vi "Teleop.vi"(10 "Match Info":T5={"Autonomous Elapsed Seconds"=0.0, "TeleOp Elapsed Seconds"=0.0, "Disabled Elapsed Seconds"=0.0, "Visited Autonomous"=FALSE, "Visited TeleOp"=FALSE, "Visited Disabled"=FALSE, "Autonomous Settings"={"Autonomous Style"=enum."Independent", "VI Refnum"=refnum}}, 11 "Call Context":T6) -> ()   [LabVIEW 2016]
doc: "This VI is called for each TeleOp packet received from the DS where the robot is not disabled. It is often used to read from the joysticks and update I/O or to update setpoints for timed control loops. It should complete and return within 20 milliseconds or it may miss DS packets."
uses:
  <vilib>/Rock Robotics/WPI/DriverStation/WPI_DriverStationDerivedRobotMode.ctl
  <vilib>/Rock Robotics/WPI/DriverStation/WPI_DriverStationMatch Info.ctl
  <vilib>/Rock Robotics/WPI/Relay/WPI_RelayValue.ctl
  <vilib>/Rock Robotics/WPI/Solenoid/WPI_SolenoidValue.ctl
  <vilib>/Rock Robotics/WPI/Utilities/WPI_GetSetVariantRefNum.vi
  <vilib>/Rock Robotics/Network Tables/NT Write Boolean Array.vi
  <vilib>/Rock Robotics/Network Tables/NT Write Numeric Array.vi
  <vilib>/Rock Robotics/Network Tables/NT Read Boolean.vi
  <vilib>/Rock Robotics/Network Tables/NT Read Number.vi
  <vilib>/Rock Robotics/WPI/Solenoid/WPI_SolenoidSetEnum.vi
  <vilib>/Rock Robotics/Network Tables/NT Write Number.vi
  Robot Global Data - Test.vi
  <vilib>/addons/control/pid/pid.llb/PID (DBL).vi
  <vilib>/Rock Robotics/WPI/RobotDrive/WPI_RobotDriveMecanumDrive_Cartesian.vi
  <vilib>/addons/control/pid/NI_PID_pid.lvlib
  <vilib>/Rock Robotics/Network Tables/NT Write Boolean.vi
panel:
  out "Relay Toggle Output":bool
  out "RelayValue":T1
  out "Compressor Running":bool
  out "Enabled":bool
  out "Raw Out Left":cluster{dbl, dbl}(graph)={0.03662109, 0.056152338}
  out "Raw Out Right":cluster{dbl, dbl}(graph)={0.0288085908, 0.026855466}
  out "Average of Right Infrared":cluster{dbl, dbl}(graph)={2232.752755466602, 2291.2959364383637}
  out "Average of Left Infrared":cluster{dbl, dbl}(graph)={1983.0102786129094, 926.8937522387996}
  out "error out":errorcluster
  out "PSI":dbl(knob) scale=0.0..200.0
  out "Average of Right Ultrasonic":cluster{dbl, dbl}(graph)={2232.752755466602, 2291.2959364383637}
  out "Average of Left Ultrasonic":cluster{dbl, dbl}(graph)={1983.0102786129094, 926.8937522387996}
  in  "climberpower":dbl(slide)=0.3 scale=0.0..1.0
  in  "deadband thing":dbl=0.13
  in  "Strafe":dbl(slide)=1.0 caption="Strafe Scale" scale=0.0..1.0
  in  "Deadband":dbl(slide)=0.10404624277456642 scale=-1.0..1.0
  out "useless data point LOL":dbl=-2.99
  out "derivative time (Td, min)":dbl
  out "integral time (Ti, min)":dbl=0.01
  out "proportional gain (Kc)":dbl=1.0
  in  "PID gains":T2={"proportional gain (Kc)"=1.0, "integral time (Ti, min)"=0.01, "derivative time (Td, min)"=0.0} {"derivative time (Td, min)" scale=0.0..0.05; "integral time (Ti, min)" scale=0.0..0.00243; "proportional gain (Kc)" scale=0.0..0.284195}
  in  "setpoint":dbl(slide) scale=-50.0..50.0
  out "Data":T3(graph)={"setpoint"=0.0, "Yaw"=-2.99, "dt out (s)"=0.018000000854954123}
  out "Yaw":dbl=-2.99
  out "YRPHfH 2":T4={"Yaw"=-2.99, "Roll"=1.62, "Pitch"=0.41, "Heading"=0.0, "Fused Heading"=357.0}
  out "Sample Slider 1":dbl(slide) scale=0.0..5.0
  out "Sample Boolean 3":bool
  out "Sample Boolean 2":bool
  in  "Match Info 2":T5={"Autonomous Elapsed Seconds"=0.0, "TeleOp Elapsed Seconds"=24.241, "Disabled Elapsed Seconds"=0.519, "Visited Autonomous"=FALSE, "Visited TeleOp"=TRUE, "Visited Disabled"=TRUE, "Autonomous Settings"={"Autonomous Style"=enum."Independent", "VI Refnum"=refnum}}
  in  "Call Context 2":T6=enum."Stop"
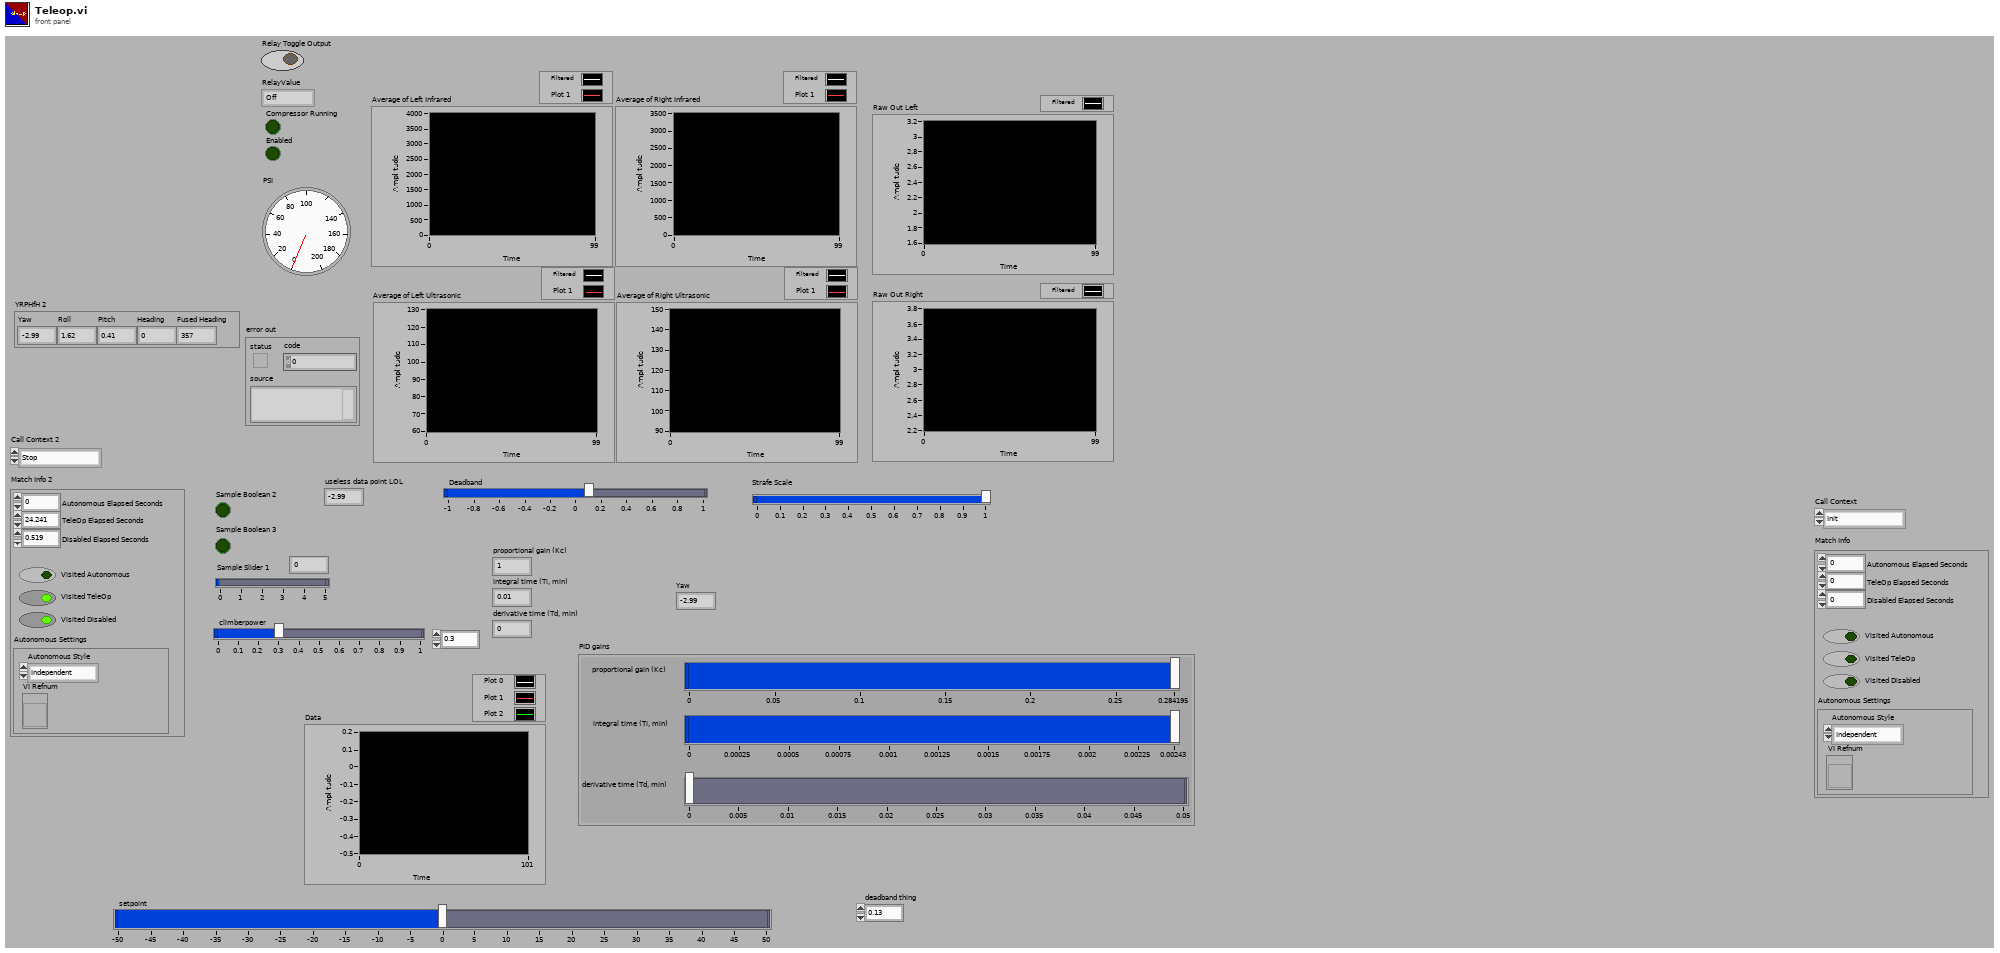
[diagram p1: front panel]
types:
  T1 = typedef "WPI_RelayValue.ctl" = enum16{"Off", "On", "Forward", "Reverse"}
  T2 = cluster{"proportional gain (Kc)":dbl, "integral time (Ti, min)":dbl, "derivative time (Td, min)":dbl}
  T3 = cluster{"setpoint":dbl, "Yaw":dbl, "dt out (s)":dbl}
  T4 = cluster{"Yaw":dbl, "Roll":dbl, "Pitch":dbl, "Heading":dbl, "Fused Heading":dbl}
  T5 = typedef "WPI_DriverStationMatch Info.ctl" = cluster{"Autonomous Elapsed Seconds":dbl, "TeleOp Elapsed Seconds":dbl, "Disabled Elapsed Seconds":dbl, "Visited Autonomous":bool, "Visited TeleOp":bool, "Visited Disabled":bool, "Autonomous Settings":cluster{"Autonomous Style":enum16{"Iterative", "Independent"}, "VI Refnum":refnum<vi>}}
  T6 = typedef "WPI_DriverStationDerivedRobotMode.ctl" = enum16{"Init", "Execute", "Stop"}
  T7 = typedef "WPI_SolenoidValue.ctl" = enum16{"Off", "On", "Forward", "Reverse"}
  T8 = typedef "WPI_AnalogChannelDevRef.ctl" = cluster{"DevStatus":errorcluster, "Analog Channel":T9}
  T9 = typedef "FPGA_AIChannel.ctl" = enum8{"AI 0", "AI 1", "AI 2", "AI 3", "AI MXP 0", "AI MXP 1", "AI MXP 2", "AI MXP 3", "Invalid"}
  T10 = typedef "WPI_CompressorDevRef.ctl" = cluster{"DevStatus":errorcluster, "Pneumatics Control Module":u8}
  T11 = typedef "WPI_RelayDevRef.ctl" = cluster{"DevStatus":errorcluster, "Relay Channel":T12, "Relay Direction":T13}
  T12 = typedef "FPGA_DIORelayChannel.ctl" = enum8{"Relay 0", "Relay 1", "Relay 2", "Relay 3", "Invalid"}
  T13 = typedef "WPI_RelayDirection.ctl" = enum16{"Both directions", "Forward only", "Reverse only"}
  T14 = typedef "WPI_JoystickDevRef.ctl" = cluster{"Device":T15}
  T15 = typedef "WPI_JoystickDeviceEnum.ctl" = enum16{"USB 0", "USB 1", "USB 2", "USB 3", "USB 4", "USB 5"}
  T16 = typedef "WPI_MotorControlDeviceRef.ctl" = cluster{"DeviceStatus":errorcluster, "Type":T17, "PWM":cluster{"PWM Channel":T18, "DeadBand":T19}, "CAN":cluster{"Device Number":u8, "SetOutput VI Ref":variant, "GetOutput VI Ref":variant, "Enable VI Ref":variant, "Disable VI Ref":variant, "Data":variant}, "Invert":bool}
  T17 = typedef "WPI_MotorControlType.ctl" = enum16{"PWM", "CAN"}
  T18 = typedef "FPGA_DIOPWMChannel.ctl" = enum8{"PWM 0", "PWM 1", "PWM 2", "PWM 3", "PWM 4", "PWM 5", "PWM 6", "PWM 7", "PWM 8", "PWM 9", "PWM MXP 0", "PWM MXP 1", "PWM MXP 2", "PWM MXP 3", "PWM MXP 4", "PWM MXP 5", "PWM MXP 6", "PWM MXP 7", "PWM MXP 8", "PWM MXP 9", "Invalid"}
  T19 = typedef "WPI_PWMDeadband.ctl" = cluster{"Name":string, "maxPositivePwm":i32, "minPositivePwm":i32, "centerPwm":i32, "maxNegativePwm":i32, "minNegativePwm":i32, "angularRange":u16}
  T20 = typedef "WPI_SolenoidDevRef.ctl" = cluster{"DevStatus":errorcluster, "Pneumatics Control Module":u8, "Forward Solenoid Channel":T21, "Reverse Solenoid Channel":T21}
  T21 = typedef "WPI_SolenoidChannel.ctl" = enum8{"Solenoid 0", "Solenoid 1", "Solenoid 2", "Solenoid 3", "Solenoid 4", "Solenoid 5", "Solenoid 6", "Solenoid 7", "Invalid"}
  T22 = typedef "WPI_RobotDriveDevRef.ctl" = cluster{"DevStatus":errorcluster, "Motors[]":T16[], "Square Inputs":bool, "Max Output":dbl}
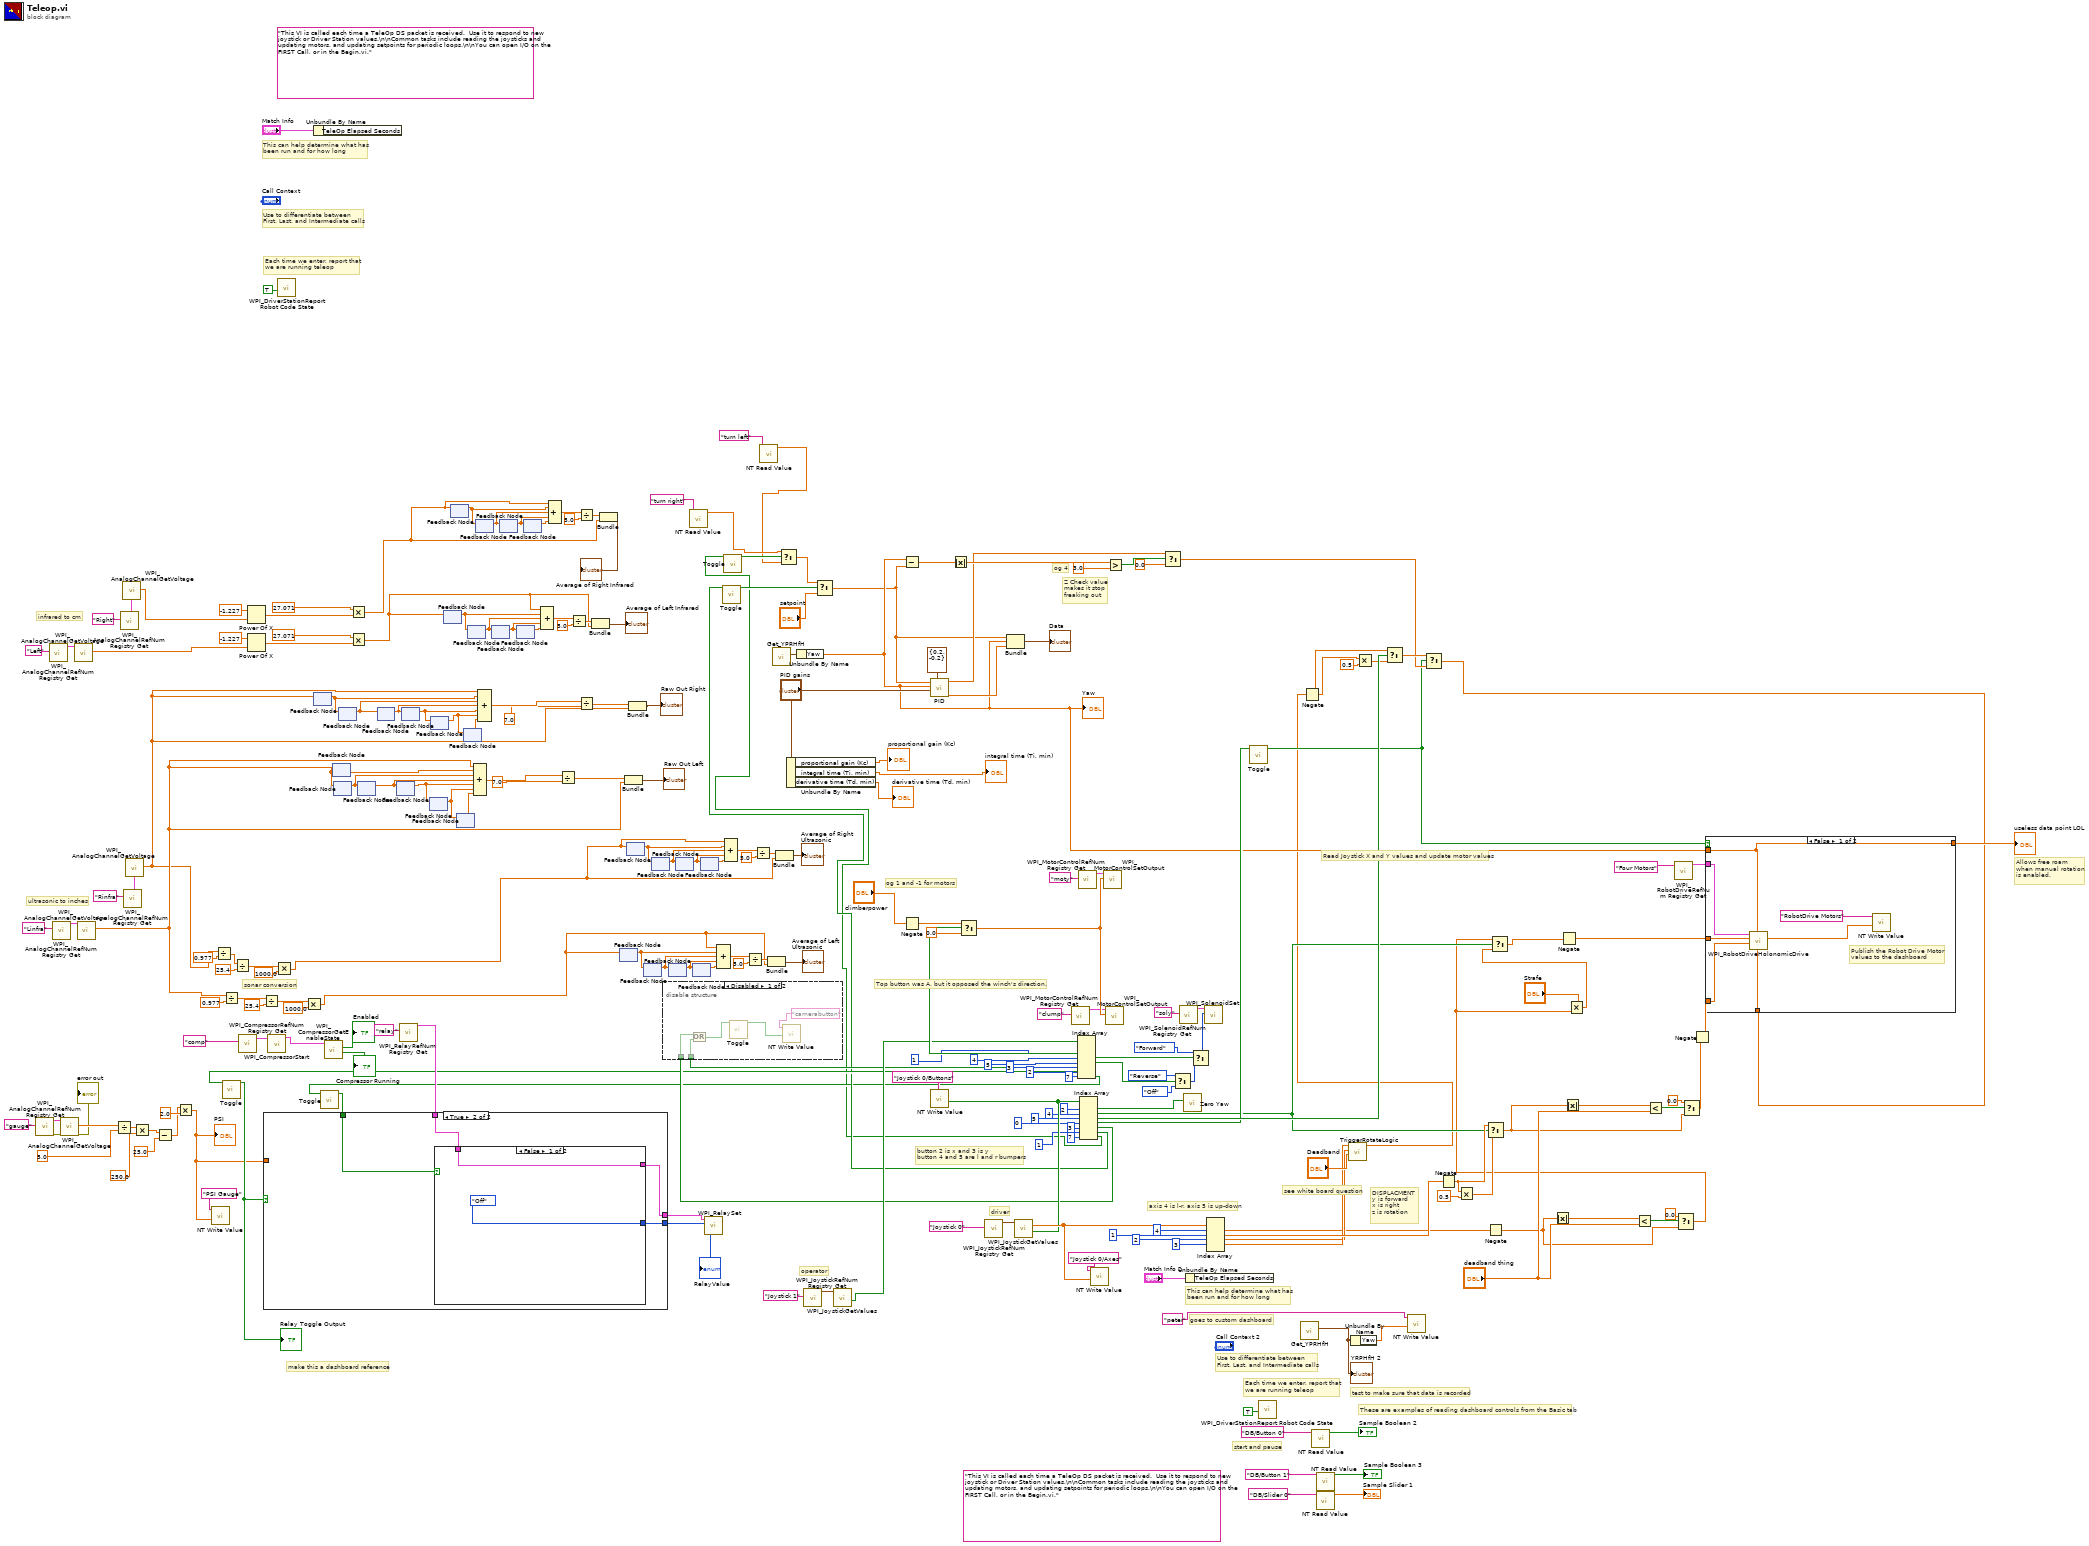
[diagram p0: block diagram]
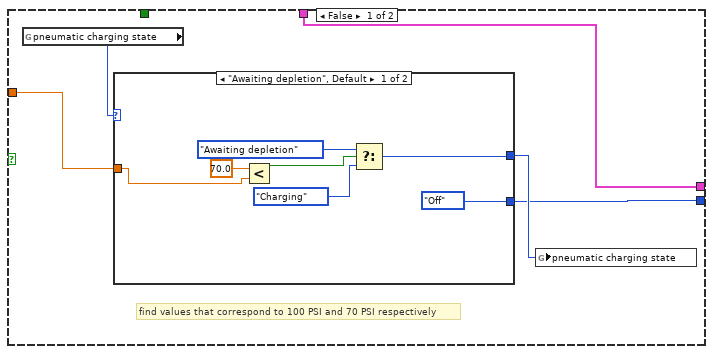
[diagram p2: hidden frame]
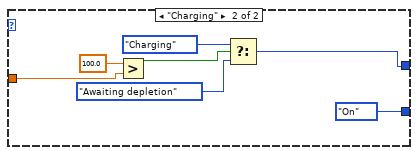
[diagram p3: hidden frame]
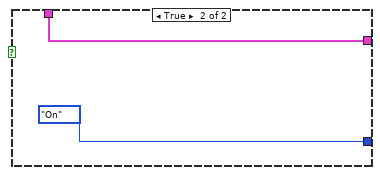
[diagram p4: hidden frame]
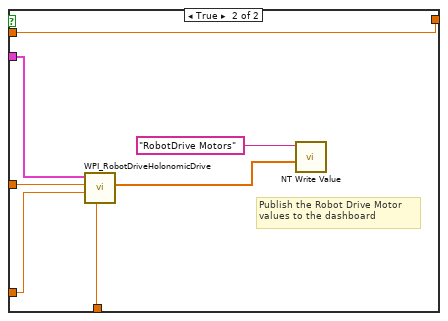
[diagram p6: hidden frame]
diagram:
  (unwired) "This VI is called each time a TeleOp DS packet is received.  Use it to respond to new joystick or Driver Station values.\n\nCommon tasks include reading the joysticks and updating motors, and updating setpoints for periodic loops.\n\nYou can open I/O on the FIRST Call, or in the Begin.vi."
  (unwired) "This VI is called each time a TeleOp DS packet is received.  Use it to respond to new joystick or Driver Station values.\n\nCommon tasks include reading the joysticks and updating motors, and updating setpoints for periodic loops.\n\nYou can open I/O on the FIRST Call, or in the Begin.vi."
  # "make this a dashboard reference"
  # "Top button was A, but it opposed the winch's direction."
  # "ultrasonic to inches"
  # "sonar conversion"
  # "infrared to cm"
  # "driver"
  # "operator"
  # "see white board question"
  # "axis 4 is l-r, axis 5 is up-down"
  # "og 1 and -1 for motors"
  # "og 4"
  # "Allows free roam\nwhen manual rotation\nis enabled."
  # "Z Check value\nmakes it stop\nfreaking out"
  # "start and pause"
  # "goes to custom dashboard"
  # "button 2 is x and 3 is y\nbutton 4 and 5 are l and r bumpers"
  # "DISPLACMENT\ny is forward\nx is right\nz is rotation"
  # "test to make sure that data is recorded"
  # "These are examples of reading dashboard controls from the Basic tab"
  # "Each time we enter, report that\nwe are running teleop"
  # "Use to differentiate between\nFirst, Last, and Intermediate calls"
  # "This can help determine what has\nbeen run and for how long"
  # "Read Joystick X and Y values and update motor values"
  # "Each time we enter, report that\nwe are running teleop"
  # "Use to differentiate between\nFirst, Last, and Intermediate calls"
  # "This can help determine what has\nbeen run and for how long"
  n1 = call <vilib>:"WPI_AnalogChannelRefNum Registry Get.vi"("refnum name"="gauge") -> ("error out"=w63:errorcluster, "AIDeviceRef"=w71:T8)  [unwired: 9 in]
  n2 = call <vilib>:"WPI_AnalogChannelRefNum Registry Get.vi"("refnum name"="Left") -> ("AIDeviceRef"=w46:T8)  [unwired: 9 in, 1 out]
  n3 = call <vilib>:"WPI_AnalogChannelRefNum Registry Get.vi"("refnum name"="Linfra") -> ("AIDeviceRef"=w128:T8)  [unwired: 9 in, 1 out]
  n4 = call <vilib>:"WPI_AnalogChannelGetVoltage.vi"("error in (no error)"=w63, "AIDeviceRef"=w71) -> ("error out"=→"error out":errorcluster, "Voltage"=w69:dbl)  [unwired: 7 in, 1 out]
  n5 = call <vilib>:"WPI_AnalogChannelGetVoltage.vi"("AIDeviceRef"=w46) -> ("Voltage"=w44:dbl)  [unwired: 8 in, 2 out]
  n6 = call <vilib>:"WPI_AnalogChannelGetVoltage.vi"("AIDeviceRef"=w128) -> ("Voltage"=w80:dbl)  [unwired: 8 in, 2 out]
  n7 = Divide(x=w69, y=5.0) -> (x/y=w68:dbl)
  n8 = call <vilib>:"WPI_AnalogChannelRefNum Registry Get.vi"("refnum name"="Right") -> ("AIDeviceRef"=w47:T8)  [unwired: 9 in, 1 out]
  n9 = call <vilib>:"WPI_AnalogChannelGetVoltage.vi"("AIDeviceRef"=w47) -> ("Voltage"=w45:dbl)  [unwired: 8 in, 2 out]
  n10 = call <vilib>:"WPI_AnalogChannelRefNum Registry Get.vi"("refnum name"="Rinfra") -> ("AIDeviceRef"=w129:T8)  [unwired: 9 in, 1 out]
  n11 = call <vilib>:"WPI_AnalogChannelGetVoltage.vi"("AIDeviceRef"=w129) -> ("Voltage"=w77:dbl)  [unwired: 8 in, 2 out]
  n12 = Multiply(x=w68, y=250.0) -> (x*y=w66:dbl)
  n13 = Subtract(x=w66, y=25.0) -> (x-y=w2:dbl)
  n14 = Multiply(x=w2, y=2.0) -> (x*y=w1:dbl)
  "PSI" <- w1
  n15 = call-poly <vilib>:"NT Write Value.vi"("Numeric"=w1, "Name"="PSI Gauge") -> ()  [unwired: 9 in, 1 out]
  n16 = Divide(x=w77, y=0.977) -> (x/y=w89:dbl)
  n17 = Divide(x=w80, y=0.977) -> (x/y=w83:dbl)
  n18 = Divide(x=w89, y=25.4) -> (x/y=w87:dbl)
  n19 = call <vilib>:"WPI_CompressorRefNum Registry Get.vi"("refnum name"="comp") -> ("CompressorDevRef"=w74:T10)  [unwired: 9 in, 1 out]
  n20 = Power Of X(1:w45, 2:-1.227 ("y")) -> (0:w41:dbl)
  n21 = Power Of X(1:w44, 2:-1.227 ("y")) -> (0:w40:dbl)
  n22 = Divide(x=w83, y=25.4) -> (x/y=w85:dbl)
  n23 = call <vilib>:"WPI_CompressorStart.vi"("CompressorDevRef"=w74) -> ("CompressorDevRef"=w6:T10)  [unwired: 9 in, 1 out]
  n24 = Multiply(x=w87, y=1000.0) -> (x*y=w81:dbl)
  n25 = call <vilib>:"WPI_DriverStationReport Robot Code State.vi"("TeleOp"=TRUE ("Autonomous")) -> ()  [unwired: 10 in, 1 out]
  n26 = Multiply(x=w85, y=1000.0) -> (x*y=w79:dbl)
  n27 = Unbundle By Name("Match Info") -> ()  [unwired: 1 out]
  n28 = feedback #1() -> (w103:dbl)  [unwired: 1 in]
  n29 = feedback-in #1(w77) -> ()
  n30 = call <vilib>:"WPI_CompressorGetEnableState.vi"("CompressorDevRef"=w6) -> ("Compressor Running"=→"Compressor Running":bool, "Enabled"=→"Enabled":bool)  [unwired: 7 in, 2 out]
  n31 = feedback #2() -> (w102:dbl)  [unwired: 1 in]
  n32 = feedback-in #2(w80) -> ()
  n33 = feedback #3() -> (w97:dbl)  [unwired: 1 in]
  n34 = feedback-in #3(w102) -> ()
  n35 = feedback #4() -> (w108:dbl)  [unwired: 1 in]
  n36 = feedback-in #4(w103) -> ()
  n37 = Multiply(x=27.071, y=w41) -> (x*y=w22:dbl)
  n38 = Multiply(x=27.071, y=w40) -> (x*y=w23:dbl)
  n39 = feedback #5() -> (w101:dbl)  [unwired: 1 in]
  n40 = feedback-in #5(w97) -> ()
  n41 = feedback #6() -> (w104:dbl)  [unwired: 1 in]
  n42 = feedback-in #6(w108) -> ()
  n43 = feedback #7() -> (w96:dbl)  [unwired: 1 in]
  n44 = feedback-in #7(w101) -> ()
  n45 = call <vilib>:"WPI_RelayRefNum Registry Get.vi"("refnum name"="relay") -> ("RelayDevRef"=w73:T11)  [unwired: 9 in, 1 out]
  n46 = feedback #8() -> (w93:dbl)  [unwired: 1 in]
  n47 = feedback-in #8(w104) -> ()
  n48 = feedback #9() -> (w95:dbl)  [unwired: 1 in]
  n49 = feedback-in #9(w96) -> ()
  n50 = feedback #10() -> (w92:dbl)  [unwired: 1 in]
  n51 = feedback-in #10(w93) -> ()
  n52 = feedback #11() -> (w37:dbl)  [unwired: 1 in]
  n53 = feedback-in #11(w23) -> ()
  n54 = feedback #12() -> (w24:dbl)  [unwired: 1 in]
  n55 = feedback-in #12(w22) -> ()
  n56 = feedback #13() -> (w94:dbl)  [unwired: 1 in]
  n57 = feedback-in #13(w95) -> ()
  n58 = feedback #14() -> (w91:dbl)  [unwired: 1 in]
  n59 = feedback-in #14(w92) -> ()
  n60 = feedback #15() -> (w36:dbl)  [unwired: 1 in]
  n61 = feedback-in #15(w37) -> ()
  n62 = Compound Arithmetic op=ADD(w80, w102, w97, w101, w96, w95, w94) -> (w98:dbl)
  n63 = feedback #16() -> (w30:dbl)  [unwired: 1 in]
  n64 = feedback-in #16(w24) -> ()
  n65 = Compound Arithmetic op=ADD(w77, w103, w108, w104, w93, w92, w91) -> (w107:dbl)
  n66 = feedback #17() -> (w31:dbl)  [unwired: 1 in]
  n67 = feedback-in #17(w36) -> ()
  n68 = feedback #18() -> (w25:dbl)  [unwired: 1 in]
  n69 = feedback-in #18(w30) -> ()
  n70 = feedback #19() -> (w32:dbl)  [unwired: 1 in]
  n71 = feedback-in #19(w31) -> ()
  n72 = feedback #20() -> (w26:dbl)  [unwired: 1 in]
  n73 = feedback-in #20(w25) -> ()
  n74 = Compound Arithmetic op=ADD(w23, w37, w36, w31, w32) -> (w35:dbl)
  n75 = Compound Arithmetic op=ADD(w22, w24, w30, w25, w26) -> (w29:dbl)
  n76 = Divide(x=w98, y=7.0) -> (x/y=w100:dbl)
  n77 = Divide(x=w35, y=5.0) -> (x/y=w33:dbl)
  n78 = Divide(x=w29, y=5.0) -> (x/y=w27:dbl)
  n79 = Divide(x=w107, y=7.0) -> (x/y=w105:dbl)
  n80 = Bundle(w33, w23) -> (→"Average of Left Infrared":cluster{dbl, dbl})  [unwired: 1 in]
  n81 = Bundle(w27, w22) -> (→"Average of Right Infrared":cluster{dbl, dbl})  [unwired: 1 in]
  n82 = feedback #21() -> (w124:dbl)  [unwired: 1 in]
  n83 = feedback-in #21(w79) -> ()
  n84 = Bundle(w100, "Voltage"=w80) -> (→"Raw Out Left":cluster{dbl, "Voltage":dbl})  [unwired: 1 in]
  n85 = feedback #22() -> (w110:dbl)  [unwired: 1 in]
  n86 = feedback-in #22(w81) -> ()
  n87 = Bundle(w105, "Voltage"=w77) -> (→"Raw Out Right":cluster{dbl, "Voltage":dbl})  [unwired: 1 in]
  n88 = feedback #23() -> (w123:dbl)  [unwired: 1 in]
  n89 = feedback-in #23(w124) -> ()
  n90 = feedback #24() -> (w116:dbl)  [unwired: 1 in]
  n91 = feedback-in #24(w110) -> ()
  n92 = feedback #25() -> (w117:dbl)  [unwired: 1 in]
  n93 = feedback-in #25(w123) -> ()
  n94 = feedback #26() -> (w111:dbl)  [unwired: 1 in]
  n95 = feedback-in #26(w116) -> ()
  n96 = call-poly <vilib>:"NT Read Value.vi"("Name"="turn right") -> ("Numeric"=w10:dbl)  [unwired: 9 in, 1 out]
  n97 = feedback #27() -> (w118:dbl)  [unwired: 1 in]
  n98 = feedback-in #27(w117) -> ()
  n99 = feedback #28() -> (w112:dbl)  [unwired: 1 in]
  n100 = feedback-in #28(w111) -> ()
  n101 = Compound Arithmetic op=ADD(w79, w124, w123, w117, w118) -> (w122:dbl)
  n102 = Compound Arithmetic op=ADD(w81, w110, w116, w111, w112) -> (w115:dbl)
  n103 = Divide(x=w122, y=5.0) -> (x/y=w120:dbl)
  n104 = Divide(x=w115, y=5.0) -> (x/y=w113:dbl)
  n105 = call-poly <vilib>:"NT Read Value.vi"("Name"="turn left") -> ("Numeric"=w9:dbl)  [unwired: 9 in, 1 out]
  n106 = Bundle(w120, w79) -> (→"Average of Left Ultrasonic":cluster{dbl, dbl})  [unwired: 1 in]
  n107 = call <vilib>:"Get_YPRHfH.vi"() -> ("YRPHfH"=w183:T4)  [unwired: 11 in]
  n108 = Bundle(w113, w81) -> (→"Average of Right Ultrasonic":cluster{dbl, dbl})  [unwired: 1 in]
  n109 = Unbundle By Name("PID gains") -> ("proportional gain (Kc)"=→"proportional gain (Kc)":dbl, "integral time (Ti, min)"=→"integral time (Ti, min)":dbl, "derivative time (Td, min)"=→"derivative time (Td, min)":dbl)
  n110 = Unbundle By Name(w183) -> ("Yaw"=w150:dbl)
  "Yaw" <- w150
  n111 = call <vilib>:"WPI_JoystickRefNum Registry Get.vi"("refnum name"="Joystick 1") -> ("JoystickDevRef"=w135:T14)  [unwired: 1 in, 9 out]
  n112 = call <vilib>:"WPI_JoystickGetValues.vi"("JoystickDevRef"=w135) -> ("Buttons"=w134:bool[])  [unwired: 6 in, 4 out]
  n113 = Negate(x="climberpower") -> (-x=w137:dbl)
  n114 = call <vilib>:"WPI_JoystickRefNum Registry Get.vi"("refnum name"="Joystick 0") -> ("JoystickDevRef"=w229:T14)  [unwired: 1 in, 9 out]
  n115 = call <vilib>:"WPI_JoystickGetValues.vi"("JoystickDevRef"=w229) -> ("Buttons"=w202:bool[], "Axes"=w226:dbl[])  [unwired: 6 in, 3 out]
  n116 = call-poly <vilib>:"NT Write Value.vi"("Boolean Array"=w202, "Name"="Joystick 0/Buttons") -> ()  [unwired: 9 in, 1 out]
  n117 = call <vilib>:"WPI_MotorControlRefNum Registry Get.vi"("refnum name"="clump") -> ("MotorControlDevRef"=w194:T16)  [unwired: 9 in, 1 out]
  n118 = Index Array(array=w134, index #2=1 ("index"), index #3=4 ("index"), index #4=5 ("index"), index #5=3 ("index"), index #6=2 ("index"), index #7=7 ("index")) -> (element #2=w215:bool, element #3=w157:bool, element #4=w155:bool, element #5=w127:bool, element #6=w56:bool, element #7=w14:bool)  [unwired: 1 in, 1 out]
  n119 = call "Toggle.vi"("Button Input"=w56) -> ("Toggle Output"=w16:bool)  [unwired: 9 in, 1 out]
  "Relay Toggle Output" <- w16
  n120 = call "Toggle.vi"("Button Input"=w14) -> ("Toggle Output"=w13:bool)  [unwired: 9 in, 1 out]
  n121 = case shown="True" w16 {
    tunnel: w73 -> [w237 w258]
    tunnel: w1 -> [w239 _]
    tunnel: w13 -> [_ w257]
    tunnel: [w237 w256] -> w8
    tunnel: [w236 w255] -> w7
    frame False {
      # "find values that correspond to 100 PSI and 70 PSI respectively"
      n122 = global read "Robot Global Data - Test.vi" "pneumatic charging state"() -> (w240:enum16{"Awaiting depletion", "Charging"})
      n123 = case shown="\"Awaiting depletion\", Default" w240 {
        tunnel: [WPI_RelayValue."Off" ("RelayValue") WPI_RelayValue."On" ("RelayValue")] -> w236
        tunnel: w239 -> [w242 w252]
        tunnel: [w241 w248] -> w238
        frame "Awaiting depletion", Default {
          n124 = Less?(x=70.0, y=w242) -> (x < y?=w245:bool)
          n125 = Select(t=enum16{"Awaiting depletion", "Charging"}."Awaiting depletion" ("pneumatic charging state"), s=w245, f=enum16{"Awaiting depletion", "Charging"}."Charging" ("pneumatic charging state")) -> (s? t:f=w241:enum16{"Awaiting depletion", "Charging"})
        }
        frame "Charging" {
          n126 = Greater?(x=100.0, y=w252) -> (0:w251:bool)
          n127 = Select(t=enum16{"Awaiting depletion", "Charging"}."Charging" ("pneumatic charging state"), s=w251, f=enum16{"Awaiting depletion", "Charging"}."Awaiting depletion" ("pneumatic charging state")) -> (s? t:f=w248:enum16{"Awaiting depletion", "Charging"})
        }
      }
      n128 = global write "Robot Global Data - Test.vi" "pneumatic charging state"(w238) -> ()
    }
    frame True {
      n129 = case shown="False" w257 {
        tunnel: w258 -> [w260 w262]
        tunnel: [w260 w262] -> w256
        tunnel: [WPI_RelayValue."Off" ("RelayValue") WPI_RelayValue."On" ("RelayValue")] -> w255
        frame False {
        }
        frame True {
        }
      }
    }
  }
  "RelayValue" <- w7
  n130 = call <vilib>:"WPI_RelaySet.vi"("RelayValue"=w7, "RelayDevRef"=w8) -> ()  [unwired: 8 in, 2 out]
  n131 = Select(t=w137, s=w215, f=0.0) -> (s? t:f=w213:dbl)
  n132 = call <vilib>:"WPI_MotorControlRefNum Registry Get.vi"("refnum name"="moty") -> ("MotorControlDevRef"=w216:T16)  [unwired: 9 in, 1 out]
  n133 = Index Array(array=w202, index #1=2 ("index"), index #2=4 ("index"), index #3=5 ("index"), index #4=0 ("index"), index #5=3 ("index"), index #6=1 ("index"), index #7=7 ("index")) -> (element #1=w152:bool, element #2=w145:bool, element #3=w198:bool, element #4=w175:bool, element #5=w126:bool, element #6=w53:bool, element #7=w11:bool)
  n134 = disable-structure shown="Disabled" {
    disable-tunnel: w127 -> [w266 _]
    disable-tunnel: w126 -> [w265 _]
    frame Disabled {
      n135 = Or(x=w265, y=w266) -> (x .or. y?=w264:bool)
      n136 = call "Toggle.vi"("Button Input"=w264) -> ("Toggle Output"=w263:bool)  [unwired: 9 in, 1 out]
      n137 = call-poly <vilib>:"NT Write Value.vi"("Boolean"=w263, "Name"="camerabutton") -> ()  [unwired: 9 in, 1 out]
    }
    frame Enabled {
    }
  }
  n138 = call "Toggle.vi"("Button Input"=w53) -> ("Toggle Output"=w52:bool)  [unwired: 9 in, 1 out]
  n139 = call "Toggle.vi"("Button Input"=w11) -> ("Toggle Output"=w54:bool)  [unwired: 9 in, 1 out]
  n140 = Select(t=w10, s=w54, f=w9) -> (s? t:f=w55:dbl)
  n141 = Select(t=w55, s=w52, f="setpoint") -> (s? t:f=w60:dbl)
  n142 = Subtract(x=w150, y=w60) -> (x-y=w187:dbl)
  n143 = call-poly <vilib>:"PID.vi"("output range"=cluster{"output high":dbl, "output low":dbl} {"output high"=0.2, "output low"=-0.2}, "PID gains"="PID gains", "process variable"=w150, "setpoint"=w60) -> ("dt out (s)"=w180:dbl, "output"=w179:dbl)  [unwired: 6 in]
  n144 = Absolute Value(x=w187) -> (abs(x)=w188:dbl)
  n145 = Bundle("setpoint"=w60, "Yaw"=w150, "dt out (s)"=w180) -> (→"Data":T3)  [unwired: 1 in]
  n146 = call-poly <vilib>:"NT Write Value.vi"("Numeric Array"=w226, "Name"="Joystick 0/Axes") -> ()  [unwired: 9 in, 1 out]
  n147 = call <vilib>:"WPI_MotorControlSetOutput.vi"("Output"=w213, "MotorControlDevRef"=w216) -> ()  [unwired: 7 in, 3 out]
  n148 = call <vilib>:"WPI_MotorControlSetOutput.vi"("Output"=w213, "MotorControlDevRef"=w194) -> ()  [unwired: 7 in, 3 out]
  n149 = Greater?(x=w188, y=3.0) -> (0:w149:bool)
  n150 = Select(t=w179, s=w149, f=0.0) -> (s? t:f=w181:dbl)
  n151 = Select(t=WPI_SolenoidValue."Reverse" ("Value"), s=w155, f=WPI_SolenoidValue."Off" ("Value")) -> (s? t:f=w158:T7)
  n152 = call <vilib>:"WPI_SolenoidRefNum Registry Get.vi"("refnum name"="soly") -> ("SolenoidDevRef"=w212:T20)  [unwired: 9 in, 1 out]
  n153 = call <vilib>:"Zero Yaw.vi"("Zero"=w152) -> ()  [unwired: 11 in]
  n154 = Unbundle By Name("Match Info 2") -> ()  [unwired: 1 out]
  n155 = Select(t=WPI_SolenoidValue."Forward" ("Value"), s=w157, f=w158) -> (s? t:f=w211:T7)
  n156 = call-poly <vilib>:"WPI_SolenoidSet.vi"("Value"=w211, "SolenoidDevRef"=w212) -> ()  [unwired: 8 in, 2 out]
  n157 = Index Array(array=w226, index #1=4 ("index"), index #2=1 ("index"), index #3=2 ("index"), index #4=3 ("index")) -> (element #1=w161:dbl, element #2=w192:dbl, element #3=w168:dbl, element #4=w169:dbl)  [unwired: 1 in, 1 out]
  n158 = call "Toggle.vi"("Button Input"=w175) -> ("Toggle Output"=w148:bool)  [unwired: 9 in, 1 out]
  n159 = call <vilib>:"WPI_DriverStationReport Robot Code State.vi"("TeleOp"=TRUE ("Autonomous")) -> ()  [unwired: 10 in, 1 out]
  n160 = call <vilib>:"Get_YPRHfH.vi"() -> ("YRPHfH"=w153:T4)  [unwired: 11 in]
  "YRPHfH 2" <- w153
  n161 = call-poly <vilib>:"NT Read Value.vi"("Name"="DB/Button 0" ("refnum name")) -> ("Boolean"=→"Sample Boolean 2":bool)  [unwired: 9 in, 1 out]
  n162 = call-poly <vilib>:"NT Read Value.vi"("Name"="DB/Slider 0" ("refnum name")) -> ("Numeric"=→"Sample Slider 1":dbl)  [unwired: 9 in, 1 out]
  n163 = call-poly <vilib>:"NT Read Value.vi"("Name"="DB/Button 1" ("refnum name")) -> ("Boolean"=→"Sample Boolean 3":bool)  [unwired: 9 in, 1 out]
  n164 = call "TriggerRotateLogic.vi"("Deadband"="Deadband", "Right Trigger"=w168, "Left Trigger"=w169) -> ("Output"=w142:dbl)  [unwired: 8 in]
  n165 = Negate(x=w142) -> (-x=w139:dbl)
  n166 = Unbundle By Name(w153) -> ("Yaw"=w204:dbl)
  n167 = Multiply(x=w139, y=0.5) -> (x*y=w197:dbl)
  n168 = Select(t=w139, s=w198, f=w197) -> (s? t:f=w182:dbl)
  n169 = call-poly <vilib>:"NT Write Value.vi"("Numeric"=w204, "Name"="peter") -> ()  [unwired: 9 in, 1 out]
  n170 = Select(t=w182, s=w148, f=w181) -> (s? t:f=w143:dbl)
  n171 = Negate(x=w192) -> (-x=w171:dbl)
  n172 = Multiply(x=w171, y=0.5) -> (x*y=w191:dbl)
  n173 = Select(t=w171, s=w145, f=w191) -> (s? t:f=w144:dbl)
  n174 = Negate(x=w161) -> (-x=w140:dbl)
  n175 = Absolute Value(x=w140) -> (abs(x)=w159:dbl)
  n176 = Absolute Value(x=w144) -> (abs(x)=w164:dbl)
  n177 = Less?(x=w159, y="deadband thing") -> (x < y?=w162:bool)
  n178 = Less?(x=w164, y="deadband thing") -> (x < y?=w167:bool)
  n179 = call <vilib>:"WPI_RobotDriveRefNum Registry Get.vi"("refnum name"="Four Motors") -> ("RobotDriveDevRef"=w231:T22)  [unwired: 1 in, 9 out]
  n180 = Select(t=0.0, s=w162, f=w140) -> (s? t:f=w141:dbl)
  n181 = Multiply(x="Strafe", y=w141) -> (x*y=w146:dbl)
  n182 = Select(t=w141, s=w145, f=w146) -> (s? t:f=w17:dbl)
  n183 = Negate(x=w17) -> (-x=w58:dbl)
  n184 = Select(t=0.0, s=w167, f=w144) -> (s? t:f=w165:dbl)
  n185 = Negate(x=w165) -> (-x=w57:dbl)
  n186 = case shown="False" w148 {
    tunnel: w231 -> [w270 w281]
    tunnel: w57 -> [w272 w278]
    tunnel: w58 -> [w271 w277]
    tunnel: w150 -> [w269 w276]
    tunnel: [w269 w276] -> w173
    tunnel: w143 -> [w268 w275]
    frame False {
      # "Publish the Robot Drive Motor\nvalues to the dashboard"
      n187 = call-poly <vilib>:"WPI_RobotDriveHolonomicDrive.vi"("Rotation"=w268, "Gyro Angle"=w269, "Y"=w272, "X"=w271, "RobotDriveDevRef"=w270) -> ("Motor Values"=w273:dbl[])  [unwired: 4 in, 2 out]
      n188 = call-poly <vilib>:"NT Write Value.vi"("Numeric Array"=w273, "Name"="RobotDrive Motors") -> ()  [unwired: 9 in, 1 out]
    }
    frame True {
      # "Publish the Robot Drive Motor\nvalues to the dashboard"
      n189 = call-poly <vilib>:"WPI_RobotDriveHolonomicDrive.vi"("Rotation"=w275, "Y"=w278, "X"=w277, "RobotDriveDevRef"=w281) -> ("Motor Values"=w279:dbl[])  [unwired: 5 in, 2 out]
      n190 = call-poly <vilib>:"NT Write Value.vi"("Numeric Array"=w279, "Name"="RobotDrive Motors") -> ()  [unwired: 9 in, 1 out]
    }
  }
  "useless data point LOL" <- w173
